vi "Agilent 2000 3000 X-Series Acquire Waveform.vi"() -> ()   [LabVIEW 2015]
doc: "This example shows how to use autosetup and acquire a waveform on a single channel."
uses:
  Agilent 2000 3000 X-Series.lvlib
panel:
  in  "Auto Scale Source (0: Channel 1)":i32(ring) items=["Channel 1"=0, "Channel 2"=1, "Channel 3"=2, "Channel 4"=3, "Digital Bus Low"=9, "Digital Bus High"=10]
  in  "Maximum Time (10000 ms)":u32=10000
  in  "Probe Attenuation (10.0)":dbl=10.0
  out "Waveform Data":waveform(dbl)(graph)
  in  "VISA resource name":refnum<visa-resource-name>
  # "(c) 2011-2023 National Instruments.  ALL RIGHTS RESERVED."
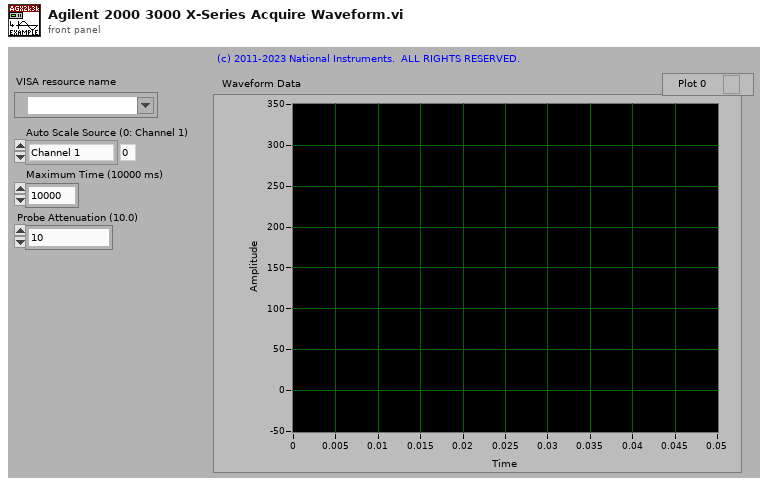
[diagram p1: front panel]
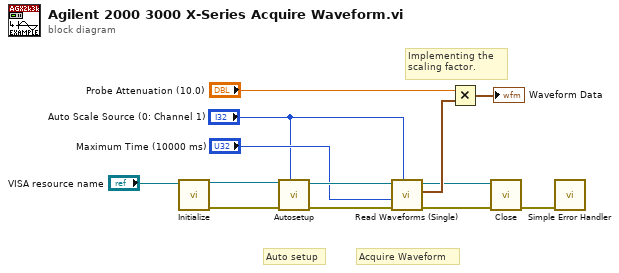
[diagram p0: block diagram]
diagram:
  # "Implementing the \nscaling factor."
  # "Acquire Waveform"
  # "Auto setup"
  n1 = call "Initialize.vi"("VISA resource name"="VISA resource name") -> ("error out"=w11:errorcluster, "VISA resource name out"=w10:refnum<visa-resource-name>)  [unwired: 4 in, 5 out]
  n2 = call "Autosetup.vi"("Auto Scale Source (0: Channel 1)"="Auto Scale Source (0: Channel 1)", "error in (no error)"=w11, "VISA resource name"=w10) -> ("error out"=w3:errorcluster, "VISA resource name out"=w4:refnum<visa-resource-name>)  [unwired: 3 in, 4 out]
  n3 = call "Read Waveforms (Single).vi"("Bind Source Channel (2: None)"="Auto Scale Source (0: Channel 1)", "error in (no error)"=w3, "Timeout (10000 ms)"="Maximum Time (10000 ms)", "VISA resource name"=w4) -> ("error out"=w7:errorcluster, "Waveform Data"=w6:waveform(dbl), "VISA resource name out"=w5:refnum<visa-resource-name>)  [unwired: 1 in, 4 out]
  n4 = Multiply(x="Probe Attenuation (10.0)", y=w6) -> (x*y=→"Waveform Data":waveform(dbl))
  n5 = call "Close.vi"("error in (no error)"=w7, "VISA resource name"=w5) -> ("error out"=w13:errorcluster)  [unwired: 9 out]
  n6 = call <vilib>:"Simple Error Handler.vi"("error in (no error)"=w13) -> ()  [unwired: 1 in, 8 out]
